vi "GyroRead.vi"(8 "Error In":errorcluster, 9 "Time Out (ms)":u32=1000, 10 "reset integrator":bool, 11 "GyroReference In":T2={"I2C Reference"={"myRIO Reference"={"myRIO Model"=enum."Unknown", "myRIO Hardware Reference"={"Generic FPGA Reference"=refnum, "Allow multiple opens"=FALSE}}, "I2C Channels Enum"=enum."Not Connected", "I2C Configuration"={"I2C Transfer Rate"=enum."Fast Mode (400 kbps)"}}, "DIO Reference"={"myRIO Reference"={"myRIO Model"=enum."Unknown", "myRIO Hardware Reference"={"Generic FPGA Reference"=refnum, "Allow multiple opens"=FALSE}}, "DIO Channels List"=[]}, "PmodGYRO address"=0}) -> (0 "Error Out":errorcluster, 1 "Angular displacement [LSB]":T1(graph), 2 "Angular rate [LSB/sec]":cluster{i16, i16, i16}(graph), 3 "GyroReference Out":T2={"I2C Reference"={"myRIO Reference"={"myRIO Model"=enum."Unknown", "myRIO Hardware Reference"={"Generic FPGA Reference"=refnum, "Allow multiple opens"=FALSE}}, "I2C Channels Enum"=enum."Not Connected", "I2C Configuration"={"I2C Transfer Rate"=enum."Fast Mode (400 kbps)"}}, "DIO Reference"={"myRIO Reference"={"myRIO Model"=enum."Unknown", "myRIO Hardware Reference"={"Generic FPGA Reference"=refnum, "Allow multiple opens"=FALSE}}, "DIO Channels List"=[]}, "PmodGYRO address"=0}, 4 "Hex DATA":u8[](array[numeric]) format="%02x")   [LabVIEW 2013]
uses:
  GyroReference.ctl
  <vilib>/myRIO/Instrument Drivers/Onboard IO/I2C/typedefs/I2C Reference.ctl
  <vilib>/myRIO/Common/Instrument Driver Framework/Utilities/typedefs/myRIO Generic Hardware Reference.ctl
  <vilib>/myRIO/Common/Instrument Driver Framework/Utilities/typedefs/Hardware Version Enum.ctl
  <vilib>/myRIO/Common/Instrument Driver Framework/Utilities/typedefs/myRIO v1.0 Reference.ctl
  <vilib>/myRIO/Common/Instrument Driver Framework/Utilities/typedefs/Generic FPGA Reference.ctl
  <vilib>/myRIO/Common/Instrument Driver Framework/myRIO v1.0/I2C/typedefs/I2C Channels Enum.ctl
  <vilib>/myRIO/Instrument Drivers/Onboard IO/I2C/typedefs/I2C Configuration.ctl
  <vilib>/myRIO/Instrument Drivers/Onboard IO/I2C/typedefs/I2C Transfer Rate.ctl
  <vilib>/myRIO/Instrument Drivers/Onboard IO/DIO/typedefs/DIO Reference.ctl
  <vilib>/myRIO/Common/Instrument Driver Framework/myRIO v1.0/DIO/typedefs/DIO Channels List.ctl
  <vilib>/myRIO/Common/Instrument Driver Framework/myRIO v1.0/DIO/typedefs/DIO Channels Enum.ctl
  <vilib>/Utility/error.llb/Error Cluster From Error Code.vi
  <vilib>/myRIO/Common/Instrument Driver Framework/myRIO v1.0/I2C/vis/myRIO v1.0 Write I2C.vi
  <vilib>/myRIO/Common/Instrument Driver Framework/myRIO v1.0/I2C/vis/myRIO v1.0 Read I2C.vi
  <vilib>/myRIO/Instrument Drivers/Onboard IO/I2C/I2C.lvlib
  <vilib>/ptbypt/NI_PtbyPt.lvlib
  <vilib>/myRIO/Instrument Drivers/Onboard IO/DIO/DIO.lvlib
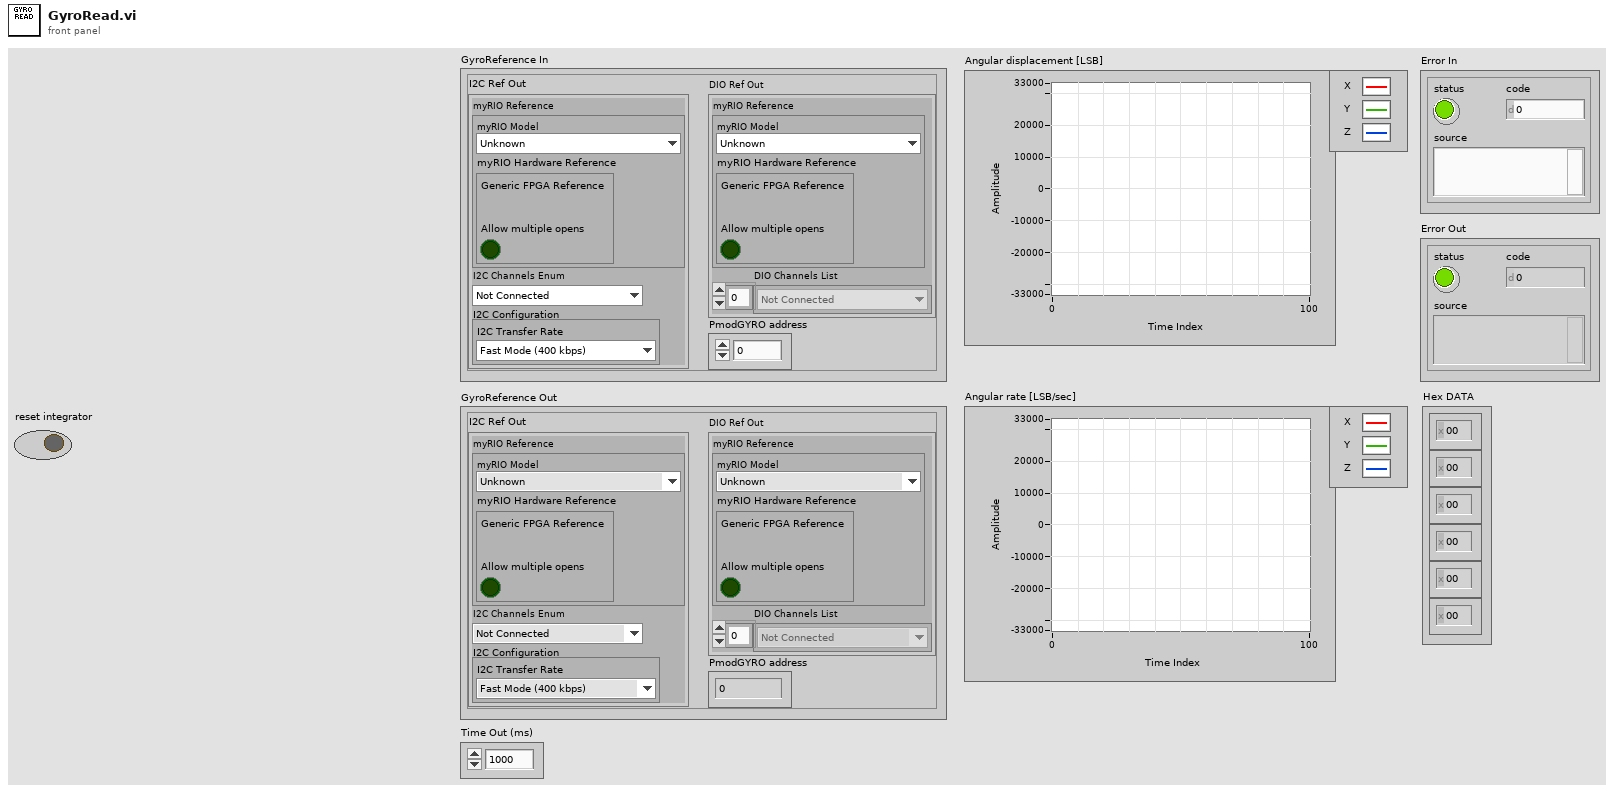
[diagram p1: front panel]
types:
  T1 = cluster{"integral x(t)":dbl, "integral x(t)":dbl, "integral x(t)":dbl}
  T2 = typedef "GyroReference.ctl" = cluster{"I2C Reference":T3, "DIO Reference":T11, "PmodGYRO address":u8}
  T3 = typedef "I2C.lvlib/I2C Reference.ctl" = cluster{"myRIO Reference":T4, "I2C Channels Enum":T8, "I2C Configuration":T9}
  T4 = typedef "myRIO Generic Hardware Reference.ctl" = cluster{"myRIO Model":T5, "myRIO Hardware Reference":T6}
  T5 = typedef "Hardware Version Enum.ctl" = enum16{"Unknown", "myRIO-1900", "myRIO-1950"}
  T6 = typedef "myRIO v1.0 Reference.ctl" = cluster{"Generic FPGA Reference":T7, "Allow multiple opens":bool}
  T7 = typedef "Generic FPGA Reference.ctl" = refnum<k20>
  T8 = typedef "I2C Channels Enum.ctl" = enum16{"Not Connected", "A/I2C", "B/I2C"}
  T9 = typedef "I2C.lvlib/I2C Configuration.ctl" = cluster{"I2C Transfer Rate":T10}
  T10 = typedef "I2C.lvlib/I2C Transfer Rate.ctl" = enum16{"Standard Mode (100 kbps)", "Fast Mode (400 kbps)"}
  T11 = typedef "DIO.lvlib/DIO Reference.ctl" = cluster{"myRIO Reference":T4, "DIO Channels List":T12}
  T12 = typedef "DIO Channels List.ctl" = T13[]
  T13 = typedef "DIO Channels Enum.ctl" = enum16{"Not Connected", "C/DIO0", "C/DIO1", "C/DIO2", "C/DIO3", "C/DIO4", "C/DIO5", "C/DIO6", "C/DIO7", "A/DIO0", "A/DIO1", "A/DIO2", "A/DIO3", "A/DIO4", "A/DIO5", "A/DIO6", "A/DIO7", "A/DIO8", "A/DIO9", "A/DIO10", "A/DIO11", "A/DIO12", "A/DIO13", "A/DIO14", "A/DIO15", "B/DIO0", "B/DIO1", "B/DIO2", "B/DIO3", "B/DIO4", "B/DIO5", "B/DIO6", "B/DIO7", "B/DIO8", "B/DIO9", "B/DIO10", "B/DIO11", "B/DIO12", "B/DIO13", "B/DIO14", "B/DIO15", "LED0", "LED1", "LED2", "LED3", "Button0"}
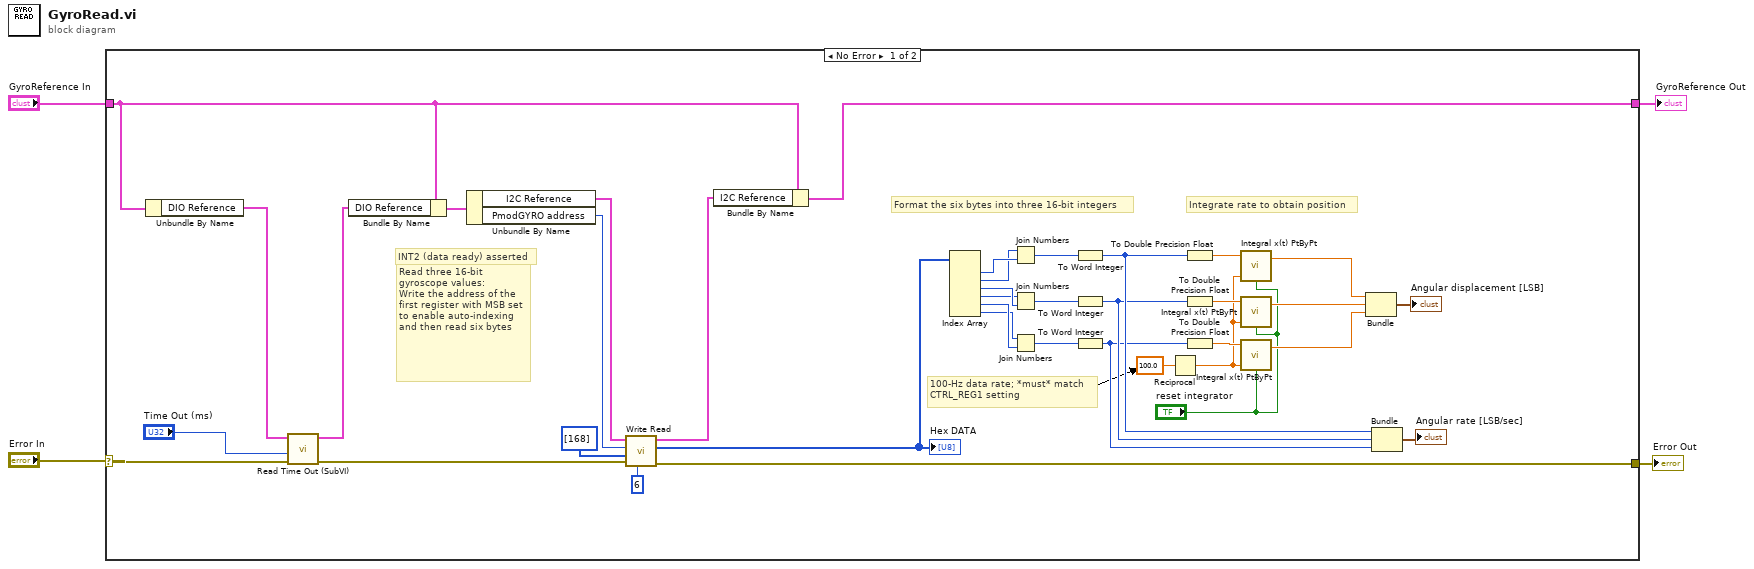
[diagram p0: block diagram]
diagram:
  n1 = case shown="No Error" "Error In" {
    selector: "Error In" -> [w42 w44]
    tunnel: "GyroReference In" -> [w8 w43]
    tunnel: [w6 w43] -> w2
    tunnel: [w40 w44] -> w1
    frame No Error {
      # "INT2 (data ready) asserted"
      # "Read three 16-bit gyroscope values:\nWrite the address of the first register with MSB set to enable auto-indexing and then read six bytes"
      # "100-Hz data rate; *must* match\nCTRL_REG1 setting"
      # "Integrate rate to obtain position"
      # "Format the six bytes into three 16-bit integers"
      n2 = Unbundle By Name(w8) -> ("DIO Reference"=w41:T11)
      n3 = call "Read Time Out (SubVI).vi"("error in (no error)"=w42, "Time Out (ms)"="Time Out (ms)", "DIO Reference"=w41) -> ("Error Out"=w12:errorcluster, "DIO Ref Out"=w13:T11)  [unwired: 7 in]
      n4 = Bundle By Name(cluster=w8, "DIO Reference"=w13) -> (w11:T2)
      n5 = Unbundle By Name(w11) -> ("I2C Reference"=w9:T3, "PmodGYRO address"=w10:u8)
      n6 = call <vilib>:"Write Read.vi"("Byte Count"=u32 6, "error in (no error)"=w12, "Bytes to Write"=u8[] [168], "Slave Address (7-bit)"=w10, "I2C Ref In"=w9) -> ("error out"=w40:errorcluster, "Bytes Read"=w27:u8[], "I2C Ref Out"=w7:T3)  [unwired: 3 in]
      "Hex DATA" <- w27
      n7 = Bundle By Name(cluster=w8, "I2C Reference"=w7) -> (w6:T2)
      n8 = Index Array "Index Array"(array=w27) -> (element #1=w35:u8, element #2=w34:u8, element #3=w33:u8, element #4=w32:u8, element #5=w31:u8, element #6=w30:u8)  [unwired: 6 in]
      n9 = Join Numbers(hi=w34, lo=w35) -> ((hi.lo)=w39:u16)
      n10 = Join Numbers(hi=w32, lo=w33) -> ((hi.lo)=w38:u16)
      n11 = Join Numbers(hi=w30, lo=w31) -> ((hi.lo)=w37:u16)
      n12 = To Word Integer(number=w39) -> (16bit integer=w26:i16)
      n13 = To Word Integer(number=w38) -> (16bit integer=w22:i16)
      n14 = To Word Integer(number=w37) -> (16bit integer=w21:i16)
      n15 = Reciprocal(x=100.0 ("dt")) -> (1/x=w19:dbl)
      n16 = To Double Precision Float(number=w26) -> (double precision float=w14:dbl)
      n17 = To Double Precision Float(number=w22) -> (double precision float=w25:dbl)
      n18 = To Double Precision Float(number=w21) -> (double precision float=w24:dbl)
      n19 = call <vilib>:"Integral x(t) PtByPt.vi"("initialize"="reset integrator", "dt"=w19, "x"=w14) -> ("integral x(t)"=w15:dbl)  [unwired: 1 in, 1 out]
      n20 = call <vilib>:"Integral x(t) PtByPt.vi"("initialize"="reset integrator", "dt"=w19, "x"=w25) -> ("integral x(t)"=w18:dbl)  [unwired: 1 in, 1 out]
      n21 = call <vilib>:"Integral x(t) PtByPt.vi"("initialize"="reset integrator", "dt"=w19, "x"=w24) -> ("integral x(t)"=w17:dbl)  [unwired: 1 in, 1 out]
      n22 = Bundle "Bundle"("integral x(t)"=w15, "integral x(t)"=w18, "integral x(t)"=w17) -> (→"Angular displacement [LSB]":T1)  [unwired: 1 in]
      n23 = Bundle "Bundle"(w26, w22, w21) -> (→"Angular rate [LSB/sec]":cluster{i16, i16, i16})  [unwired: 1 in]
    }
    frame Error {
    }
  }
  "Error Out" <- w1
  "GyroReference Out" <- w2
